vi "Write to Spreadsheet Quick.vi"(3 "2D data":sgl[][](array[numeric]) format="%0.2f", 5 "file path":path) -> ()   [LabVIEW 2017, in "File IO.lvclass"]
uses:
  File IO.lvclass
  <vilib>/Utility/file.llb/Write To Spreadsheet File (DBL).vi
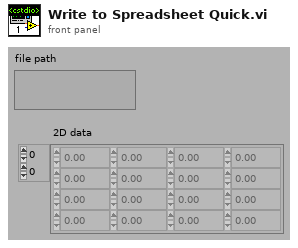
[diagram p1: front panel]
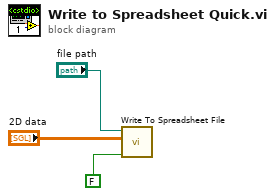
[diagram p0: block diagram]
diagram:
  n1 = call-poly <vilib>:"Write To Spreadsheet File.vi"("append to file? (new file:F)"=FALSE, "2D data"="2D data", "file path (dialog if empty)"="file path") -> ()  [unwired: 3 in, 3 out]
